vi "Scale Encoder IP to Array Index (Relative (FLR]).vi"(7 "Micropulse # In":i32, 9 "Inspection Point Location":u32, 10 "Scan definition":T1 {"Inspection Resolution" format="%#_6f"; "Scan Length" format="%#_6f"}, 11 "Axis No.":u8=1 min=1 max=4) -> (3 "B-Scan index":i32)   [LabVIEW 2026, in "MicroPulse_Driver.lvlib"]
uses:
  MicroPulse_Driver.lvlib
  Data/Datatypes/MP - fly scan range (relative).ctl
  Data/Datatypes/MP - inspection direction (relative).ctl
  <instrlib>/Micropulse/Micropulse.lvlib
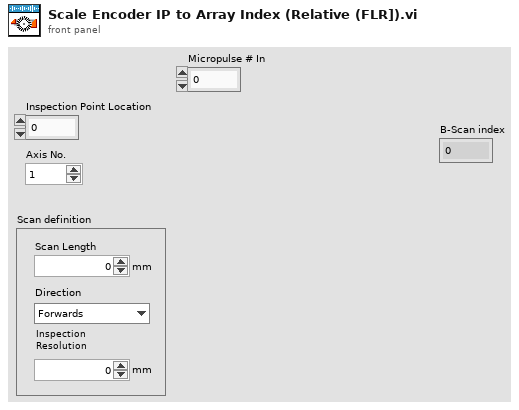
[diagram p1: front panel]
types:
  T1 = typedef "Micropulse.lvlib/MP - fly scan range (relative).ctl" = cluster{"Scan Length":dbl, "Inspection Resolution":dbl, "Direction":T2}
  T2 = typedef "Micropulse.lvlib/MP - inspection direction (relative).ctl" = enum16{"Forwards", "Backwards", "Bidirectional"}
  T3 = typedef "Micropulse.lvlib/MP-Registry Data-Cluster.ctl" = cluster{"Instrument Type":T4, "Serial #":u64, "Sample Frequency":T5, "dt (us)":dbl, "DOF":T6, "Material Velocity":dbl, "Asynch Reads":T7, "NUM of Tests":u32, "System Details":T8, "Gates":T10[], "Encoders":T17[], "CMD LUT":variant, "Command List":string}
  T4 = typedef "Micropulse.lvlib/MP - instrument type.ctl" = enum16{"MicroPulse 5", "LT1", "LT2", "LTPA", "MPLT", "MicroPulse 6", "PipeScanner", "<MicroPulse>", "Micropulse 4", "Simulated Data"}
  T5 = typedef "Micropulse.lvlib/MP - sample frequency.ctl" = enum16{"Use Default", "200MHz (LT2 only)", "100MHz", "50MHz", "25MHz", "10MHz"}
  T6 = typedef "Micropulse.lvlib/MP - data output format.ctl" = enum16{"", "8-bit Mode", "10-bit Mode", "12-bit Mode", "16-bit Mode", "8-bit Log Mode", "12-bit Packed Mode"}
  T7 = typedef "Micropulse.lvlib/MP - asynch read mode.ctl" = enum16{"Disabled", "Enabled"}
  T8 = typedef "Micropulse.lvlib/MP - general system status.ctl" = cluster{"System Type":T4, "Serial No.":u64, "Channels":cluster{"Conv":u8, "PA":u16, "Extra":u32}, "Sample Frequency":cluster{"Default":u8, "Actual":u8}, "Software Versions":string, "Data Output Format":cluster{"Default":T6, "Actual":T6}, "Temperatures":cluster{"System":u8, "Processor":u8, "Slave Sys":u8, "Slave Proc":u8}, "Tx Buffer Size":u32, "System Error":string, "No. of Cards":u8, "DAC Gain":i16, "Uptimes":cluster{"since Power":u32, "since RSTS":u32, "since SRST":u32}, "Voltages":cluster{"Nominal":dbl, "Measured":dbl, "Difference":dbl}[], "Interface Cards":T9[]}
  T9 = typedef "Micropulse.lvlib/MP - interface card status.ctl" = cluster{"Status":u8, "Map":u8, "Board - T":u8, "FPGA - T":u8, "PAIF Status":string, "Version":string}
  T10 = typedef "Micropulse.lvlib/MP - Registry Gates.ctl" = cluster{"Display Gate":T11, "ETM Mode":T12, "Echo Gate":T13, "Insp Gates":T14[]}
  T11 = typedef "Micropulse.lvlib/MP - display gate.ctl" = cluster{"Start":dbl, "Length":dbl}
  T12 = typedef "Micropulse.lvlib/MP - echo gate mode.ctl" = enum16{"Echo Trigger OFF", "Echo Gate Display Mode", "Echo Trigger ON", "Multi Gate or FMC Mode", "Reserved", "PA - Echo Trigger ON"}
  T13 = typedef "Micropulse.lvlib/MP - echo gate parameters.ctl" = cluster{"Start (us)":dbl, "Length (us)":dbl, "Threshold":u16, "Colour":u32}
  T14 = typedef "Micropulse.lvlib/MP - multigate inspection gate parameters.ctl" = cluster{"Start (us)":dbl, "Length (us)":dbl, "Threshold":u16, "Enabled?":bool, "Max # Peaks":u16, "Hysteresis":T15, "Mode":T16, "Inverted?":bool, "Colour ":u32}
  T15 = typedef "Micropulse.lvlib/MP - hysteresis level.ctl" = enum16{"None", "3dB", "6dB", "9dB", "12dB"}
  T16 = typedef "Micropulse.lvlib/MP - multigate mode.ctl" = enum16{"1st Peak in Gate", "Largest Peak In Gate", "All Peaks In Gate", "1st Threshold Crossing"}
  T17 = typedef "Micropulse.lvlib/MP - encoder settings.ctl" = cluster{"Encoder Type":T18, "Counts/mm":u32, "Enable Termination?":bool, "Multiplier":u32, "Backlash Period (s)":dbl, "Encoder Filter":u32}
  T18 = typedef "Micropulse.lvlib/MP - encoder type.ctl" = enum16{"Quadrature", "Step/Direction"}
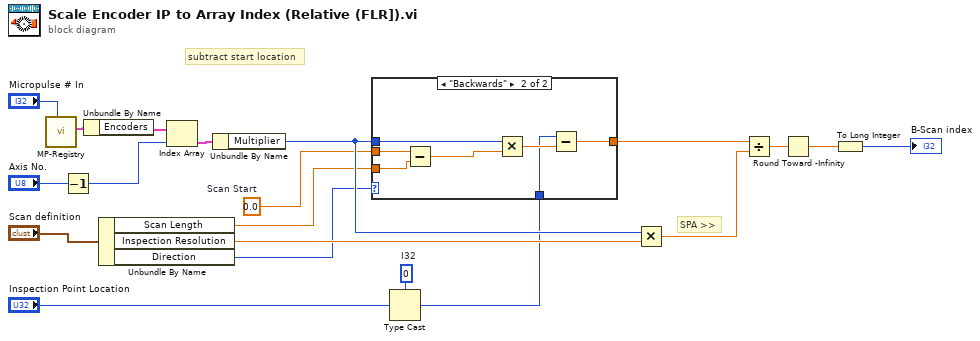
[diagram p0: block diagram]
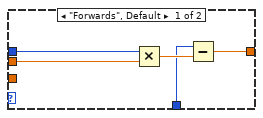
[diagram p2: hidden frame]
diagram:
  w3 = 0.0  # Scan Start
  w4 = 0  # I32
  # "subtract start location"
  # "SPA >>"
  n1 = call "MP-Registry.vi"("Micropulse # In"="Micropulse # In") -> ("Micropulse Data"=w15:T3)  [unwired: 7 in, 3 out]
  n2 = Decrement(x="Axis No.") -> (x-1=w1:u8)
  n3 = Unbundle By Name(w15) -> ("Encoders"=w14:T17[])
  n4 = Unbundle By Name("Scan definition") -> ("Scan Length"=w6:dbl, "Inspection Resolution"=w20:dbl, "Direction"=w7:T2)
  n5 = Index Array(array=w14, index=w1) -> (element=w13:T17)
  n6 = Unbundle By Name(w13) -> ("Multiplier"=w8:u32)
  n7 = Type Cast(type=w4, x="Inspection Point Location") -> (*(type *) &x=w5:i32)
  n8 = case shown="\"Backwards\"" w7 {
    tunnel: w3 -> [w25 w32]
    tunnel: w5 -> [w23 w30]
    tunnel: [w22 w29] -> w10
    tunnel: w8 -> [w21 w28]
    tunnel: w6 -> [_ w26]
    frame "Forwards", Default {
      n9 = Multiply(x=w21, y=w25) -> (x*y=w24:dbl)
      n10 = Subtract(x=w23, y=w24) -> (x-y=w22:dbl)
    }
    frame "Backwards" {
      n11 = Subtract(x=w32, y=w26) -> (x-y=w27:dbl)
      n12 = Multiply(x=w28, y=w27) -> (x*y=w31:dbl)
      n13 = Subtract(x=w30, y=w31) -> (x-y=w29:dbl)
    }
  }
  n14 = Multiply(x=w8, y=w20) -> (x*y=w12:dbl)
  n15 = Divide(x=w10, y=w12) -> (x/y=w16:dbl)
  n16 = Round Toward -Infinity(1:w16) -> (0:w9:dbl)
  n17 = To Long Integer(number=w9) -> (32bit integer=→"B-Scan index":i32)
